vi "PH_Beckhoff.get SE.vi"(0 "Sonderklemmen Inputs":T1, 1 "index of element":i32) -> (2 "DIM value":u32, 3 "Quality":bool, 4 "Tag not found":bool)   [LabVIEW 2014, in "PH_Beckhoff.lvlib"]
uses:
  PH_Beckhoff.lvlib
  PH_Beckhoff.Sonderklemmen Inputs.ctl
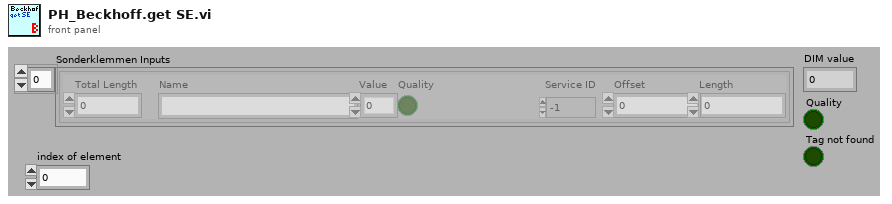
[diagram p1: front panel]
types:
  T1 = typedef "PH_Beckhoff.lvlib/PH_Beckhoff.Sonderklemmen Inputs.ctl" = cluster{"Total Length":u32, "Name":string, "Value":u64, "Quality":bool, "Service ID":i32, "Offset":u32, "Length":u32}[]
  T2 = cluster{"Total Length":u32, "Name":string, "Value":u64, "Quality":bool, "Service ID":i32, "Offset":u32, "Length":u32}
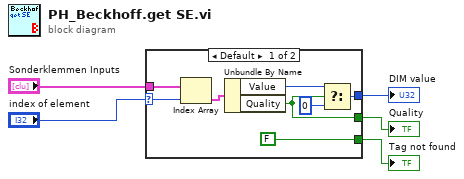
[diagram p0: block diagram]
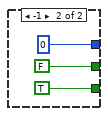
[diagram p2: hidden frame]
diagram:
  n1 = case shown="Default" "index of element" {
    selector: "index of element" -> [w11 _]
    tunnel: [w9 FALSE] -> w3
    tunnel: [w8 u32 0 ("DIM value")] -> w2
    tunnel: "Sonderklemmen Inputs" -> [w13 _]
    tunnel: [FALSE TRUE] -> w5
    frame Default {
      n2 = Index Array(array=w13, index=w11) -> (element=w12:T2)
      n3 = Unbundle By Name(w12) -> ("Value"=w6:u64, "Quality"=w9:bool)
      n4 = Select(t=w6, s=w9, f=u32 0) -> (s? t:f=w8:u64)
    }
    frame -1 {
    }
  }
  "Tag not found" <- w5
  "Quality" <- w3
  "DIM value" <- w2
